vi "intervalo.vi"(9 "Intervalo":dbl, 10 "Final":dbl, 11 "inicio":dbl) -> (2 "Array":dbl[](array[numeric]))   [LabVIEW 2016]
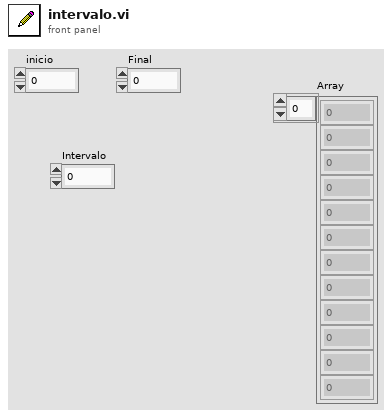
[diagram p1: front panel]
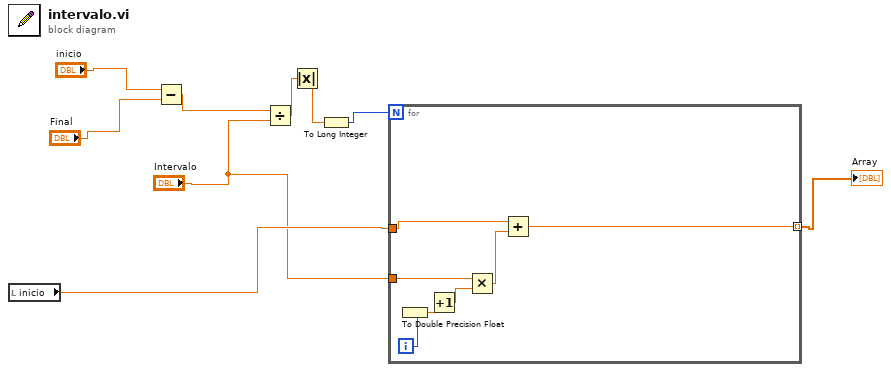
[diagram p0: block diagram]
diagram:
  n1 = local read "inicio"() -> (w6:dbl)
  n2 = Subtract(x="inicio", y="Final") -> (x-y=w7:dbl)
  n3 = Divide(x=w7, y="Intervalo") -> (x/y=w3:dbl)
  n4 = Absolute Value(x=w3) -> (abs(x)=w2:dbl)
  n5 = To Long Integer(number=w2) -> (32bit integer=w1:i32)
  n6 = for {
    N: w1 -> [_]
    tunnel: w6 -> [w15]
    tunnel: "Intervalo" -> [w16]
    tunnel: [w13] -> w4 mode=indexing
    i -> [w10]
    n7 = To Double Precision Float(number=w10) -> (double precision float=w11:dbl)
    n8 = Increment(x=w11) -> (x+1=w12:dbl)
    n9 = Multiply(x=w16, y=w12) -> (x*y=w14:dbl)
    n10 = Add(x=w15, y=w14) -> (x+y=w13:dbl)
  }
  "Array" <- w4
